vi "AI-Freq.vi"(6 "Slot":T1, 7 "DAQConfigRef":T2, 8 "error in":errorcluster, 10 "Mode":string, 11 "CH":string) -> (0 "error out":errorcluster, 3 "波形图":waveform(dbl)(graph))   [LabVIEW 2013]
uses:
  Controls/DAQConfigRef.ctl
  Controls/DAQConfig.ctl
  SystemCode/SysControl/Slot.ctl
  <vilib>/DAQmx/read.llb/DAQmx Read (Analog Wfm 1Chan NSamp).vi
  <vilib>/DAQmx/create/channels.llb/DAQmx Create Channel (AI-Voltage-Basic).vi
  <vilib>/DAQmx/configure/timing.llb/DAQmx Timing (Sample Clock).vi
  <vilib>/measure/matone.llb/Extract Single Tone Information 1 Chan.vi
  <vilib>/DAQmx/miscellaneous.llb/DAQmx Fill In Error Info.vi
  <vilib>/measure/NI_MAPro.lvlib
panel:
  out "detected frequency":dbl caption="检测到的频率" format="%.2p"
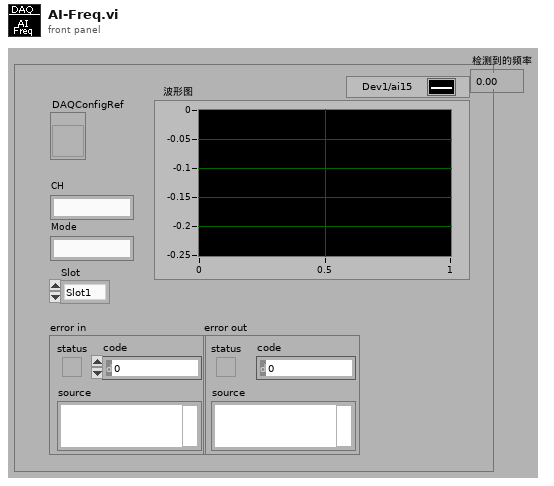
[diagram p1: front panel]
types:
  T1 = typedef "Slot.ctl" = enum16{"Slot1", "Slot2", "Slot3", "Slot4"}
  T2 = typedef "DAQConfigRef.ctl" = refnum<vi>
  T3 = typedef "DAQConfig.ctl" = cluster{"DIO":string[][], "AO":string[][], "AI":string[][]}
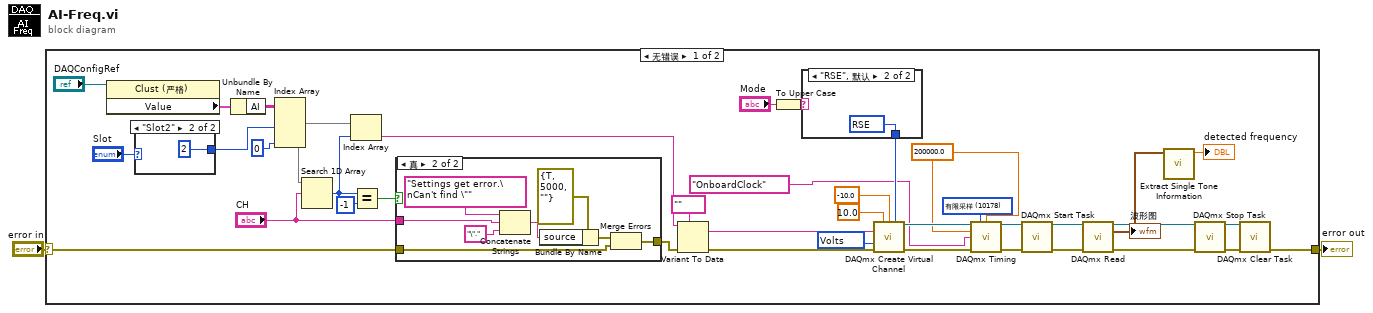
[diagram p0: block diagram]
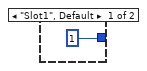
[diagram p2: hidden frame]
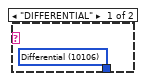
[diagram p4: hidden frame]
diagram:
  n1 = case shown="无错误" "error in" {
    selector: "error in" -> [w31 w56]
    tunnel: [w42 w56] -> w2
    frame No Error {
      w3 = 200000.0 ("rate")
      w27 = 10178 items=["有限采样"=10178, "连续采样"=10123, "硬件定时单点"=12522] ("sample mode")
      w37 = 10348 items=["Volts"=10348, "From Custom Scale"=10065] ("units")
      n2 = property class="Clust (严格)"(reference="DAQConfigRef") -> ("Value"=w17:T3)  [unwired: 1 in, 2 out]
      n3 = case shown="\"Slot2\"" "Slot" {
        tunnel: [1 ("索引 (行)") 2 ("索引 (行)")] -> w4
        frame "Slot1", Default {
        }
        frame "Slot2" {
        }
      }
      n4 = Unbundle By Name(w17) -> ("AI"=w21:string[][])
      n5 = Index Array(array=w21, index (col) #1=w4, index (col) #2=0 ("索引 (列)")) -> (element #1=w16:string[], element #2=w15:string[])  [unwired: 2 in]
      n6 = Search 1D Array(1D array=w15, element="CH") -> (index of element=w19:i32)  [unwired: 1 in]
      n7 = Index Array(array=w16, index=w19) -> (element=w9:string)
      n8 = Equal?(x=w19, y=-1) -> (x = y?=w13:bool)
      n9 = case shown="真" w13 {
        tunnel: w31 -> [w45 w48]
        tunnel: [w45 w47] -> w10
        tunnel: "CH" -> [_ w46]
        frame False {
        }
        frame True {
          n10 = Concatenate Strings("Settings get error.\nCan't find \"" ("message"), w46, "\"." ("string")) -> (w52:string)
          n11 = Bundle By Name(cluster=errorcluster {"status"=TRUE, "code"=5000, "source"=""} ("error in 1 (no error)"), "source"=w52) -> (w51:errorcluster)
          n12 = Merge Errors(w51, w48) -> (w47:errorcluster)
        }
      }
      n13 = Variant To Data(error in=w10, type=tag "" ("lines"), Variant=w9) -> (data=w33:tag, error out=w32:errorcluster)
      n14 = To Upper Case(1:"Mode") -> (0:w29:string)
      n15 = case shown="\"RSE\", 默认" w29 {
        tunnel: [w54 w55] -> w28
        frame "DIFFERENTIAL" {
          w54 = 10106 items=["default"=-1, "RSE"=10083, "NRSE"=10078, "Differential"=10106, "Pseudodifferential"=12529] ("input terminal configuration")
        }
        frame "RSE", Default {
          w55 = 10083 items=["default"=-1, "RSE"=10083, "NRSE"=10078, "Differential"=10106, "Pseudodifferential"=12529] ("input terminal configuration")
        }
      }
      n16 = call-poly <vilib>:"DAQmx Create Virtual Channel.vi"("maximum value"=10.0, "minimum value"=-10.0, "input terminal configuration"=w28, "physical channels"=w33, "units"=w37, "error in"=w32) -> ("task out"=w26:refnum<k21>, "error out"=w24:errorcluster)  [unwired: 8 in]
      n17 = call-poly <vilib>:"DAQmx Timing.vi"("task/channels in"=w26, "sample mode"=w27, "samples per channel"=w3, "rate"=w3, "source"=tag "OnboardClock" ("采样时钟源"), "error in"=w24) -> ("task out"=w25:refnum<k21>, "error out"=w23:errorcluster)  [unwired: 1 in, 7 out]
      n18 = call <vilib>:"DAQmx Start Task.vi"("task/channels in"=w25, "error in"=w23) -> ("task out"=w41:refnum<k21>, "error out"=w40:errorcluster)  [unwired: 12 in]
      n19 = call-poly <vilib>:"DAQmx Read.vi"("task/channels in"=w41, "error in"=w40) -> ("task out"=w36:refnum<k21>, "data"=w7:waveform(dbl), "error out"=w22:errorcluster)  [unwired: 11 in]
      "波形图" <- w7
      n20 = call-poly <vilib>:"Extract Single Tone Information.vi"("time signal in"=w7) -> ("detected frequency"=→"detected frequency":dbl)  [unwired: 5 in, 5 out]
      n21 = call <vilib>:"DAQmx Stop Task.vi"("task/channels in"=w36, "error in"=w22) -> ("task out"=w39:refnum<k21>, "error out"=w38:errorcluster)  [unwired: 12 in]
      n22 = call <vilib>:"DAQmx Clear Task.vi"("task in"=w39, "error in"=w38) -> ("error out"=w42:errorcluster)  [unwired: 13 in]
    }
    frame Error {
    }
  }
  "error out" <- w2
